vi "Tip Cleaner.vi"() -> ()   [LabVIEW 2021]
doc: "Moves the tip to a specfied locations and performs Bias pulses there. Useful to try to clean the tip without affecting the sample at the current position.\n\n- Nanonis Programming Interface -"
uses:
  Nanonis Prog Interface.lvlib
panel:
  in  "Pause (s)":dbl=0.02 format="%#_6p"
  in  "Feedback":enum16{"no change", "hold", "don't hold"}(ring)=enum."hold"
  out "oCleanTip":refnum<k4>
  out "AllQuit":bool=TRUE
  in  "Quit":bool
  in  "# Pulses":u16=5 min=1
  in  "CleanTip":bool
  in  "Voltage (V)":dbl=2.0 format="%_4p"
  in  "Duration (s)":dbl=0.02 format="%#_6p"
  in  "Position Y (m)":sgl=3.5e-09 format="%#_6p"
  in  "Position X (m)":sgl=-1.3e-09 format="%#_6p"
  in  "Get Tip Position":bool
  # "Cleaning Parameters"
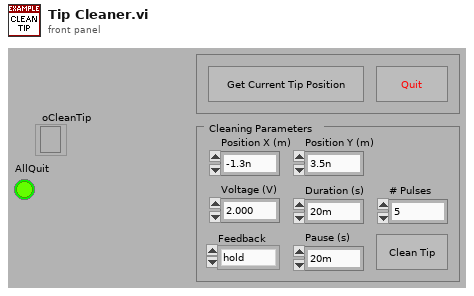
[diagram p1: front panel]
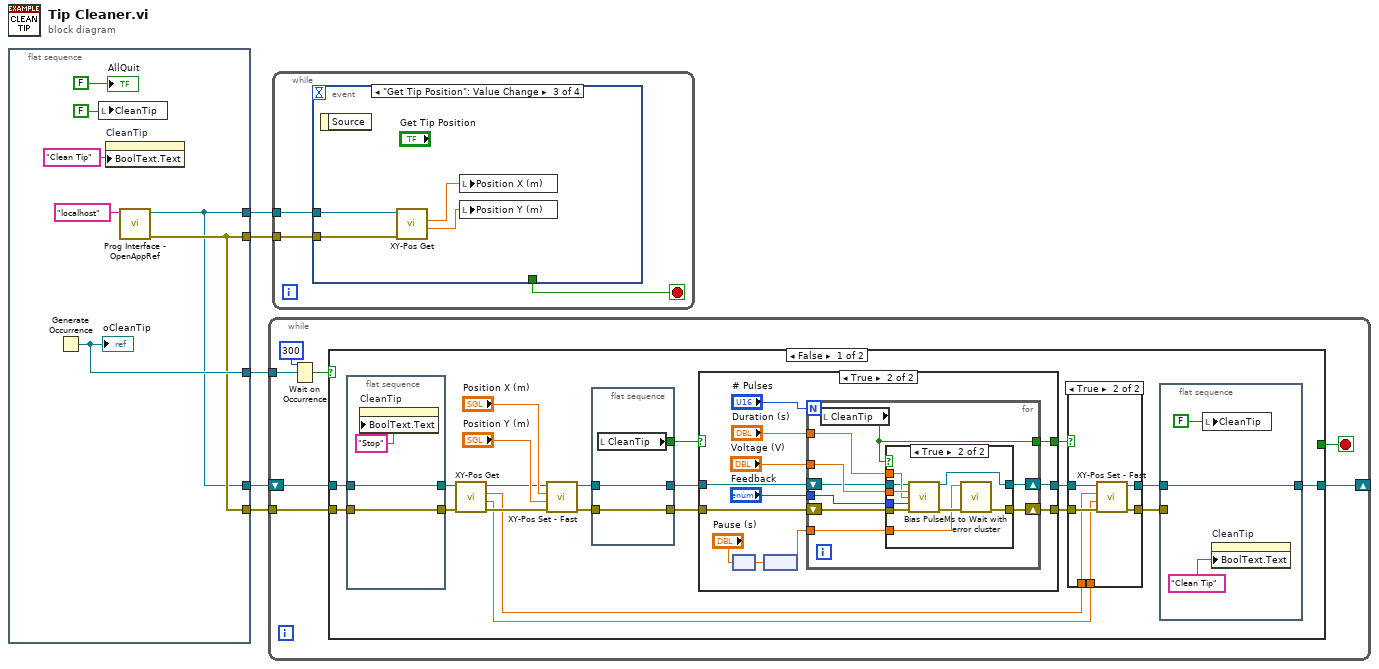
[diagram p0: block diagram]
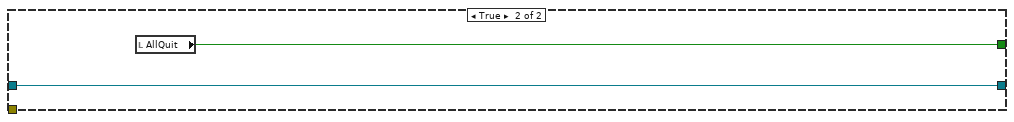
[diagram p5: hidden frame]
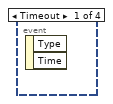
[diagram p6: hidden frame]
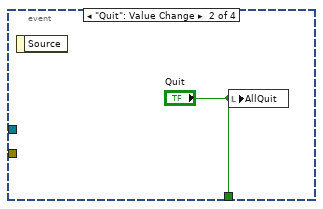
[diagram p7: hidden frame]
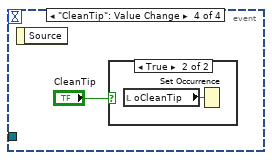
[diagram p8: hidden frame]
diagram:
  n1 = flat-sequence {
    tunnel: [w9] -> w5
    tunnel: [w7] -> w4
    tunnel: [w7] -> w3
    tunnel: [w6] -> w2
    tunnel: [w6] -> w1
    frame #0 {
      n2 = Generate Occurrence() -> (w9:refnum<k4>)
      "oCleanTip" <- w9
      n3 = local write "CleanTip"(FALSE) -> ()
      n4 = property on="CleanTip" class="Bool (strict)"("BoolText.Text"="Clean Tip" ("Boolean Text.Text")) -> ()  [unwired: 2 in, 2 out]
      n5 = call <userlib>:"Prog Interface - OpenAppRef.vi"("Machine name (local machine IP)"="localhost") -> ("Error out"=w7:errorcluster, "Application reference"=w6:refnum<vi>)  [unwired: 5 in]
      "AllQuit" <- FALSE
    }
  }
  n6 = while {
    tunnel: w5 -> [w17]
    tunnel: w4 -> [w15]
    shift-right: [w13] -> _
    shift-left: w2 -> [w14]
    stop <- w19 stop-if-true
    n7 = Wait on Occurrence(2:w17, 3:300) -> (0:w18:bool)  [unwired: 1 in]
    n8 = case shown="False" w18 {
      tunnel: [_ w94] -> w19
      tunnel: w15 -> [w34 _]
      tunnel: w14 -> [w26 w93]
      tunnel: [w20 w93] -> w13
      frame False {
        n9 = flat-sequence {
          tunnel: w34 -> [w42]
          tunnel: [w42] -> w33
          tunnel: w26 -> [w41]
          tunnel: [w41] -> w25
          frame #0 {
            n10 = property on="CleanTip" class="Bool (strict)"("BoolText.Text"="Stop" ("Boolean Text.Text")) -> ()  [unwired: 2 in, 2 out]
          }
        }
        n11 = call <userlib>:"XY-Pos Get.vi"("error in (no error)"=w33, "Application ref in"=w25) -> ("error out"=w40:errorcluster, "Y (m)"=w29:sgl, "X (m)"=w28:sgl, "Application ref out"=w27:refnum<vi>)  [unwired: 5 in]
        n12 = call <userlib>:"XY-Pos Set - Fast.vi"("error in (no error)"=w40, "Y (m)"="Position Y (m)", "X (m)"="Position X (m)", "Application ref in"=w27) -> ("error out"=w37:errorcluster, "Application ref out"=w24:refnum<vi>)  [unwired: 5 in]
        n13 = flat-sequence {
          tunnel: [w46] -> w36
          tunnel: w37 -> [w46]
          tunnel: [w45] -> w35
          tunnel: w24 -> [w44]
          tunnel: [w44] -> w23
          frame #0 {
            n14 = local read "CleanTip"() -> (w45:bool)
          }
        }
        n15 = case shown="True" w35 {
          selector: w35 -> [w56 _]
          tunnel: [w57 w69] -> w39
          tunnel: w36 -> [w57 w68]
          tunnel: [w56 w63] -> w32
          tunnel: w23 -> [w55 w59]
          tunnel: [w55 w58] -> w22
          frame False {
          }
          frame True {
            n16 = node("Pause (s)") -> (w62:dbl[unit])
            n17 = node(w62) -> (w60:dbl)
            n18 = for {
              N: "# Pulses" -> [_]
              shift-right: [w74] -> w69
              shift-left: w68 -> [w78]
              tunnel: "Feedback" -> [w77]
              tunnel: "Voltage (V)" -> [w76]
              tunnel: "Duration (s)" -> [w75]
              tunnel: [w72] -> w63
              tunnel: w60 -> [w73]
              shift-right: [w70] -> w58
              shift-left: w59 -> [w71]
              n19 = local read "CleanTip"() -> (w72:bool)
              n20 = case shown="True" w72 {
                tunnel: w78 -> [w80 w89]
                tunnel: w77 -> [_ w88]
                tunnel: w76 -> [_ w87]
                tunnel: w75 -> [_ w86]
                tunnel: [w80 w84] -> w74
                tunnel: w73 -> [_ w83]
                tunnel: w71 -> [w79 w82]
                tunnel: [w79 w81] -> w70
                frame False {
                }
                frame True {
                  n21 = call <userlib>:"Bias Pulse.vi"("Application ref in"=w82, "Pulse bias (V) (1)"=w87, "Pulse width (s) (100m)"=w86, "Z-Controller (no change)"=w88, "Error in (no error)"=w89) -> ("Application ref out"=w81:refnum<vi>, "Error out"=w85:errorcluster)  [unwired: 9 in]
                  n22 = call "Ms to Wait with error cluster.vi"("error in (no error)"=w85, "milliseconds to wait"=w83) -> ("error out"=w84:errorcluster)  [unwired: 4 in, 1 out]
                }
              }
            }
          }
        }
        n23 = case shown="True" w32 {
          tunnel: w39 -> [w48 w54]
          tunnel: [w48 w53] -> w38
          tunnel: w28 -> [_ w51]
          tunnel: w29 -> [_ w52]
          tunnel: w22 -> [w47 w50]
          tunnel: [w47 w49] -> w21
          frame False {
          }
          frame True {
            n24 = call <userlib>:"XY-Pos Set - Fast.vi"("error in (no error)"=w54, "Y (m)"=w52, "X (m)"=w51, "Application ref in"=w50) -> ("error out"=w53:errorcluster, "Application ref out"=w49:refnum<vi>)  [unwired: 5 in]
          }
        }
        n25 = flat-sequence {
          tunnel: w38 -> [_]
          tunnel: w21 -> [w90]
          tunnel: [w90] -> w20
          frame #0 {
            n26 = local write "CleanTip"(FALSE ("CleanTip")) -> ()
            n27 = property on="CleanTip" class="Bool (strict)"("BoolText.Text"="Clean Tip" ("Boolean Text.Text")) -> ()  [unwired: 2 in, 2 out]
          }
        }
      }
      frame True {
        n28 = local read "AllQuit"() -> (w94:bool)
      }
    }
  }
  n29 = while {
    tunnel: w3 -> [w96]
    tunnel: w1 -> [w95]
    stop <- w97 stop-if-true
    n30 = event shown="[2] \"Get Tip Position\": Value Change" {
      selector: _ -> [_ _ _ _]
      dyn-events: _ -> [_ _ _ _]
      timeout: _ -> [_ _ _ _]
      tunnel: [_ "Quit" _ _] -> w97
      tunnel: w96 -> [_ _ w102 _]
      tunnel: w95 -> [_ _ w99 _]
      event Timeout {
        n31 = event-data() -> ()  [unwired: 1 in, 2 out]
      }
      event "Quit": Value Change {
        n32 = event-data() -> ()  [unwired: 1 in, 1 out]
        n33 = local write "AllQuit"("Quit") -> ()
      }
      event "Get Tip Position": Value Change {
        n34 = event-data() -> ()  [unwired: 1 in, 1 out]
        n35 = call <userlib>:"XY-Pos Get.vi"("error in (no error)"=w102, "Application ref in"=w99) -> ("Y (m)"=w101:sgl, "X (m)"=w100:sgl)  [unwired: 5 in, 2 out]
        n36 = local write "Position X (m)"(w100) -> ()
        n37 = local write "Position Y (m)"(w101) -> ()
      }
      event "CleanTip": Value Change {
        n38 = event-data() -> ()  [unwired: 1 in, 1 out]
        n39 = case shown="True" "CleanTip" {
          frame False {
          }
          frame True {
            n40 = local read "oCleanTip"() -> (w104:refnum<k4>)
            n41 = Set Occurrence(w104) -> ()
          }
        }
      }
    }
  }
